vi "createEvents.vi"(8 "error in (no error)":errorcluster, 11 "MonoPubSubData in":refnum<class "MonoPubSubData.lvclass">) -> (0 "error out":errorcluster, 3 "MonoPubSubData out":refnum<class "MonoPubSubData.lvclass">)   [LabVIEW 2016, in "MonoPubSubData.lvclass"]
uses:
  MonoPubSubData.lvclass
  Typedefs/slit.ctl
  Typedefs/SlitType.ctl
  Typedefs/slitWidth.ctl
  Typedefs/GratingType.ctl
  Typedefs/wavelength.ctl
  Typedefs/DeviceStatus.ctl
  Typedefs/AckType.ctl
  MonoPubSubData.lvclass/MonoPubSubData.ctl
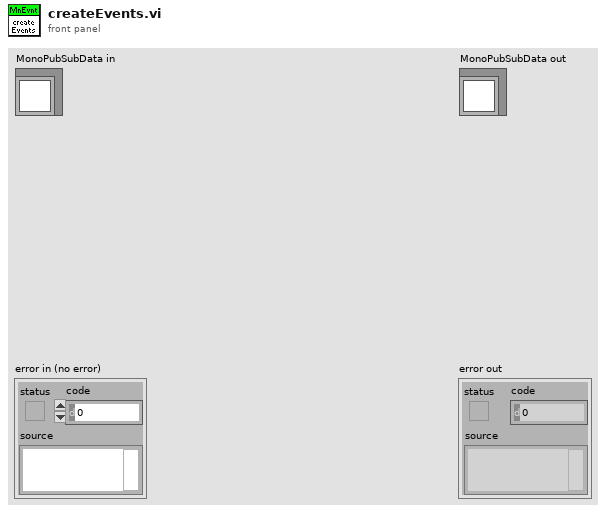
[diagram p1: front panel]
types:
  T1 = typedef "AckType.ctl" = enum16{"OK", "OutOfRange", "Unknown", "Busy", "Rejected"}
  T2 = typedef "SlitType.ctl" = enum16{"Front Entrance", "Side Entrance", "Front Exit", "Side Exit", "First Intermediate", "Second Intermediate"}
  T3 = typedef "wavelength.ctl" = dbl
  T4 = typedef "slit.ctl" = cluster{"SlitType":T2, "Width":T5}
  T5 = typedef "slitWidth.ctl" = dbl
  T6 = typedef "GratingType.ctl" = enum16{"NoGrating", "Red", "Blue", "Mirror"}
  T7 = typedef "DeviceStatus.ctl" = enum16{"SettingUp", "Ready", "Offline", "Fault"}
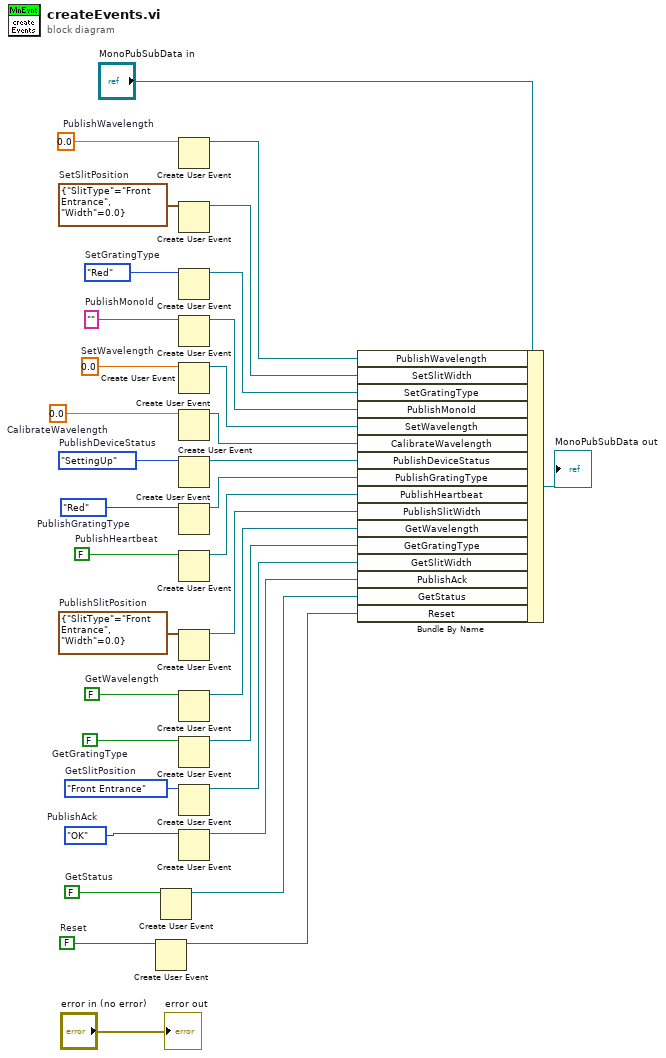
[diagram p0: block diagram]
diagram:
  w2 = FALSE  # Reset
  w4 = FALSE  # GetStatus
  w6 = AckType."OK"  # PublishAck
  w8 = SlitType."Front Entrance"  # GetSlitPosition
  w11 = FALSE  # GetWavelength
  w12 = FALSE  # GetGratingType
  w25 = T3 0.0  # PublishWavelength
  w26 = ""  # PublishMonoId
  w27 = FALSE  # PublishHeartbeat
  w28 = T4 {"SlitType"=enum."Front Entrance", "Width"=0.0}  # PublishSlitPosition
  w29 = GratingType."Red"  # PublishGratingType
  w30 = DeviceStatus."SettingUp"  # PublishDeviceStatus
  w31 = T3 0.0  # CalibrateWavelength
  w32 = T3 0.0  # SetWavelength
  w33 = GratingType."Red"  # SetGratingType
  w34 = T4 {"SlitType"=enum."Front Entrance", "Width"=0.0}  # SetSlitPosition
  n1 = Create User Event(user event datatype=w2) -> (user event=w1:refnum<user-event>)  [unwired: 1 in, 1 out]
  n2 = Create User Event(user event datatype=w4) -> (user event=w3:refnum<user-event>)  [unwired: 1 in, 1 out]
  n3 = Create User Event(user event datatype=w25) -> (user event=w19:refnum<user-event>)  [unwired: 1 in, 1 out]
  n4 = Create User Event(user event datatype=w34) -> (user event=w15:refnum<user-event>)  [unwired: 1 in, 1 out]
  n5 = Create User Event(user event datatype=w33) -> (user event=w14:refnum<user-event>)  [unwired: 1 in, 1 out]
  n6 = Create User Event(user event datatype=w26) -> (user event=w20:refnum<user-event>)  [unwired: 1 in, 1 out]
  n7 = Create User Event(user event datatype=w32) -> (user event=w17:refnum<user-event>)  [unwired: 1 in, 1 out]
  n8 = Create User Event(user event datatype=w31) -> (user event=w16:refnum<user-event>)  [unwired: 1 in, 1 out]
  n9 = Create User Event(user event datatype=w30) -> (user event=w18:refnum<user-event>)  [unwired: 1 in, 1 out]
  n10 = Create User Event(user event datatype=w29) -> (user event=w13:refnum<user-event>)  [unwired: 1 in, 1 out]
  n11 = Create User Event(user event datatype=w27) -> (user event=w21:refnum<user-event>)  [unwired: 1 in, 1 out]
  n12 = Create User Event(user event datatype=w28) -> (user event=w22:refnum<user-event>)  [unwired: 1 in, 1 out]
  n13 = Create User Event(user event datatype=w11) -> (user event=w10:refnum<user-event>)  [unwired: 1 in, 1 out]
  n14 = Create User Event(user event datatype=w12) -> (user event=w9:refnum<user-event>)  [unwired: 1 in, 1 out]
  n15 = Create User Event(user event datatype=w8) -> (user event=w7:refnum<user-event>)  [unwired: 1 in, 1 out]
  n16 = Create User Event(user event datatype=w6) -> (user event=w5:refnum<user-event>)  [unwired: 1 in, 1 out]
  n17 = Bundle By Name(cluster="MonoPubSubData in", "PublishWavelength"=w19, "SetSlitWidth"=w15, "SetGratingType"=w14, "PublishMonoId"=w20, "SetWavelength"=w17, "CalibrateWavelength"=w16, "PublishDeviceStatus"=w18, "PublishGratingType"=w13, "PublishHeartbeat"=w21, "PublishSlitWidth"=w22, "GetWavelength"=w10, "GetGratingType"=w9, "GetSlitWidth"=w7, "PublishAck"=w5, "GetStatus"=w3, "Reset"=w1) -> (→"MonoPubSubData out":refnum<class "MonoPubSubData.lvclass">)
  "error out" <- "error in (no error)"
